vi "4-5.vi"() -> ()   [LabVIEW 2017]
panel:
  in  "指定值":dbl
  out "循环次数":i32
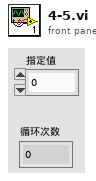
[diagram p1: front panel]
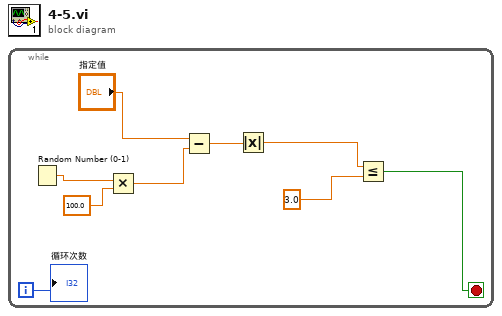
[diagram p0: block diagram]
diagram:
  n1 = while {
    i -> [w7]
    stop <- w1 stop-if-true
    n2 = Random Number (0-1) ("随机数(1-100)")() -> (number: 0 to 1=w9:dbl)
    n3 = Multiply(x=w9, y=100.0) -> (x*y=w5:dbl)
    n4 = Subtract(x="指定值", y=w5) -> (x-y=w4:dbl)
    n5 = Absolute Value(x=w4) -> (abs(x)=w3:dbl)
    n6 = Less Or Equal?(x=w3, y=3.0) -> (x <= y?=w1:bool)
    "循环次数" <- w7
  }
